vi "Test Control Experiment Dictionary.vi"() -> ()   [LabVIEW 2016]
uses:
  <userlib>/LevyLab/LV to ITX/Data/Typedefs/Dictionary--cluster.ctl
  src/Control Experiment/Control Experiment.lvclass
  <userlib>/LevyLab/LV to ITX/Data/Data.lvclass
panel:
  in  "CLOSE":bool
  out "multiple writes (ms)":u32
  out "one write (ms)":u32
  in  "TEST SPEED":bool
  in  "Append Element":cluster{"Key":string, "Value":dbl[]}
  out "Read All Items":T1[](array[typedef])
  in  "READ":bool
  in  "APPEND":bool
  in  "WRITE":bool
  in  "OK":bool
  in  "Write Element":cluster{"Key":string, "Value":dbl}
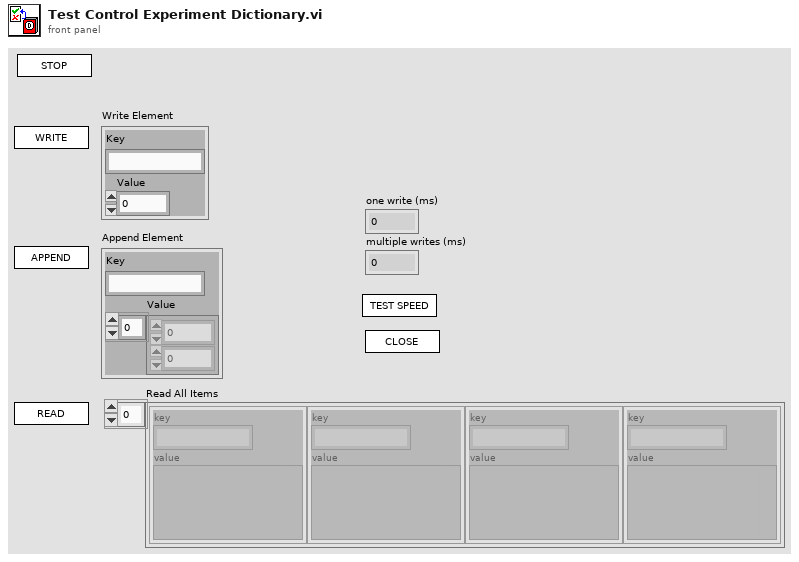
[diagram p1: front panel]
types:
  T1 = typedef "Data.lvclass/Dictionary--cluster.ctl" = cluster{"key":string, "value":variant}
  T2 = enum32{"Invalid", "Standard", "Closed", "Hidden", "Minimized", "Maximized"}
  T3 = enum32{"invalid app kind", "Development System", "Run Time System", "Student Edition", "Embedded LabVIEW", "Evaluation", "Custom"}
  T4 = cluster{"Core":cluster{"Current VI Reference":refnum<vi>, "Close Panel on Exit?":bool}, "Your Boolean data":bool, "Your string data":string, "Control Experiment.lvclass":refnum<class "Control Experiment.lvclass">}
  T5 = cluster{"Current VI Reference":refnum<vi>, "Close Panel on Exit?":bool}
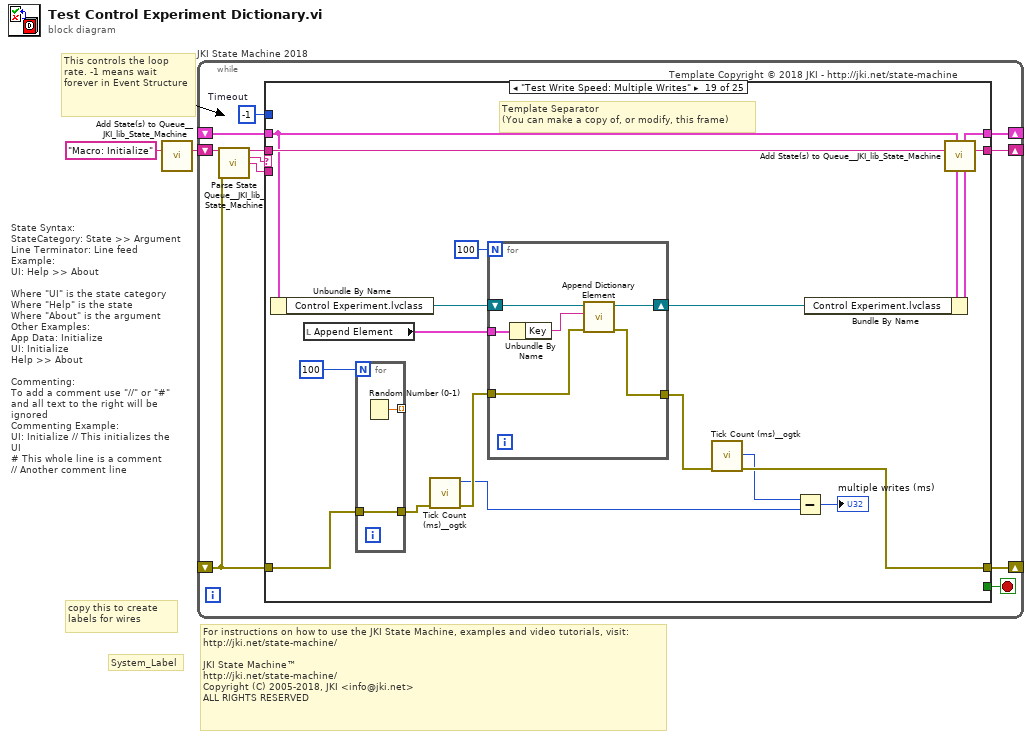
[diagram p0: block diagram]
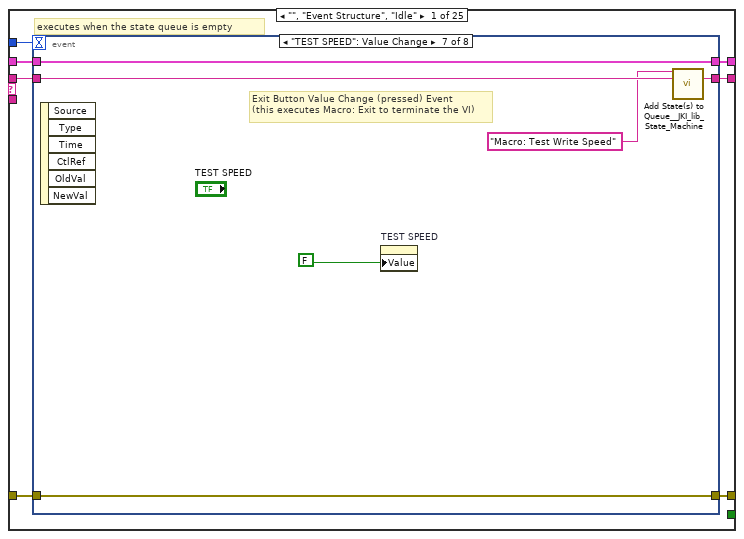
[diagram p2: hidden frame]
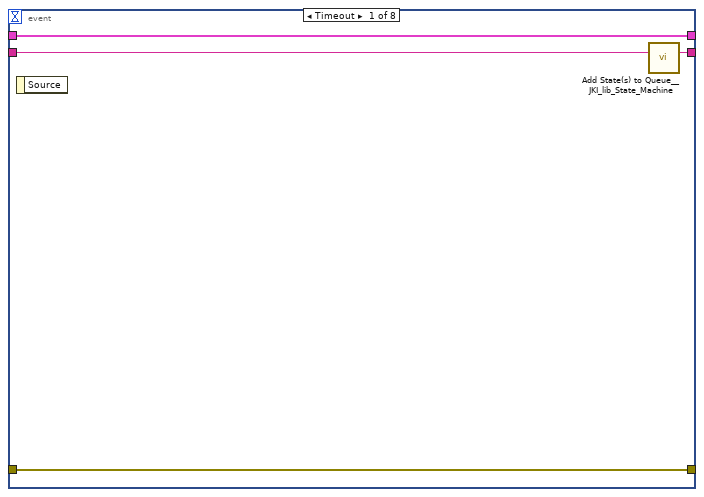
[diagram p3: hidden frame]
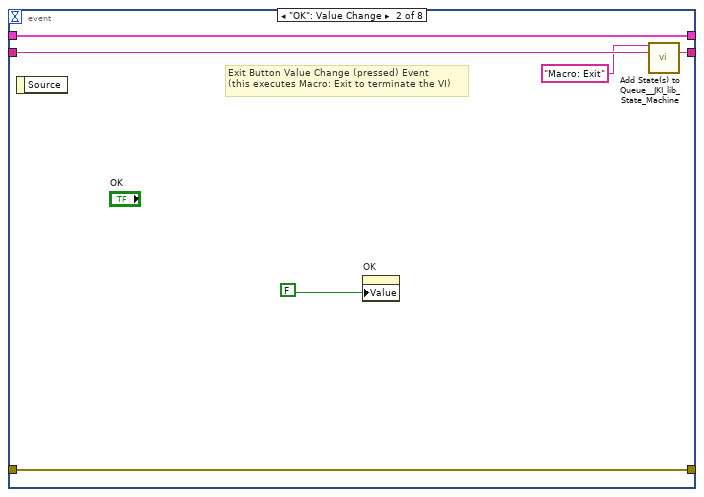
[diagram p4: hidden frame]
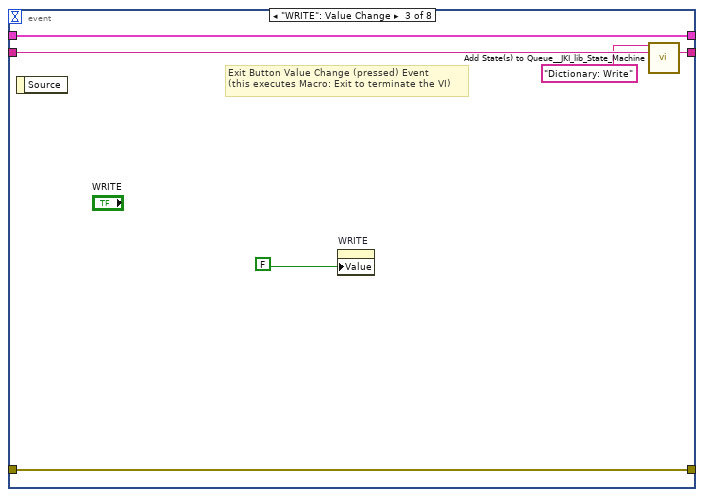
[diagram p5: hidden frame]
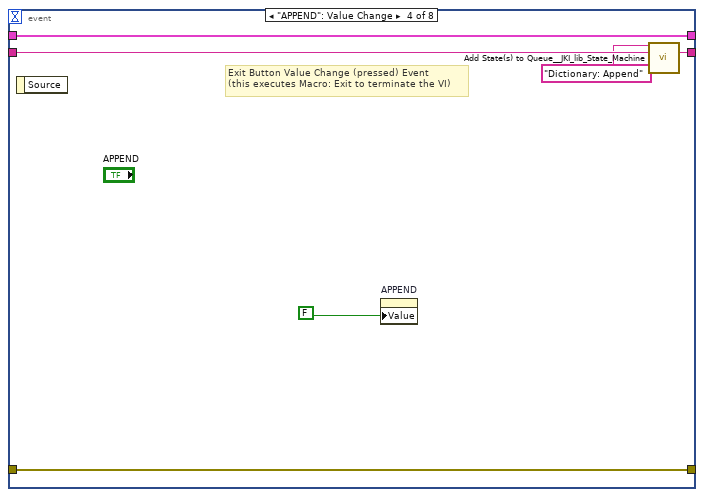
[diagram p6: hidden frame]
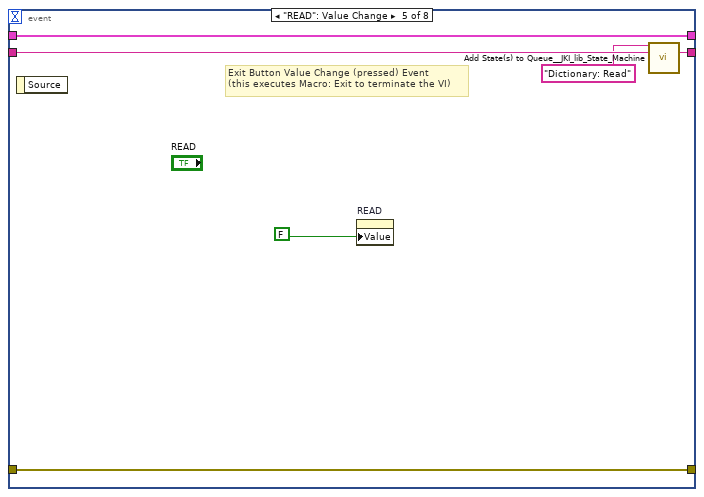
[diagram p7: hidden frame]
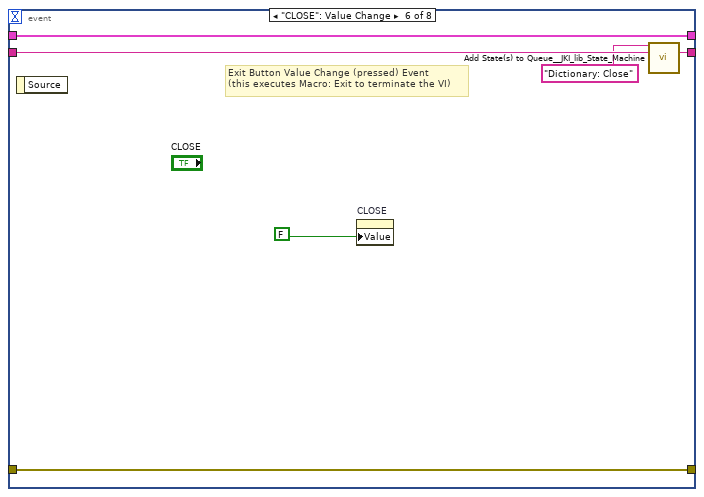
[diagram p8: hidden frame]
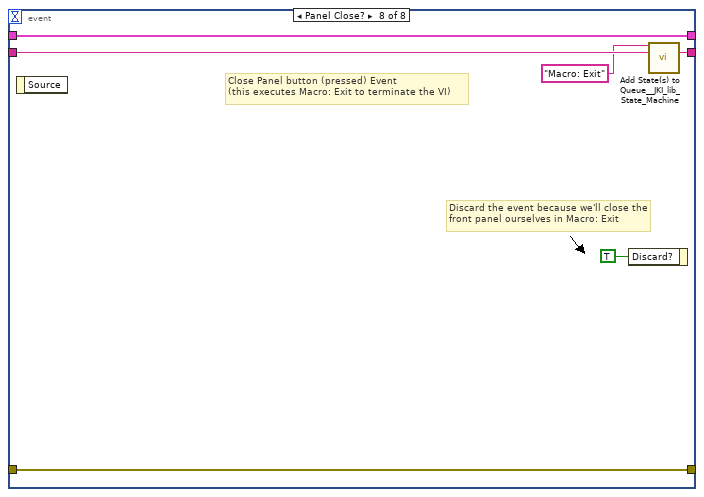
[diagram p9: hidden frame]
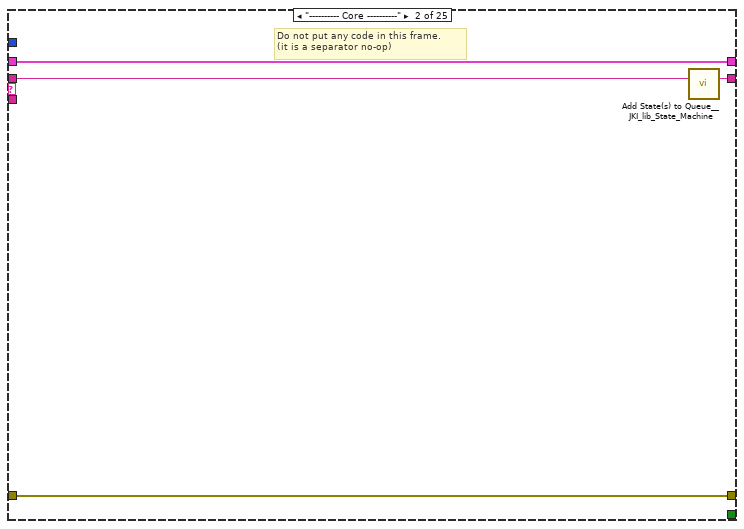
[diagram p10: hidden frame]
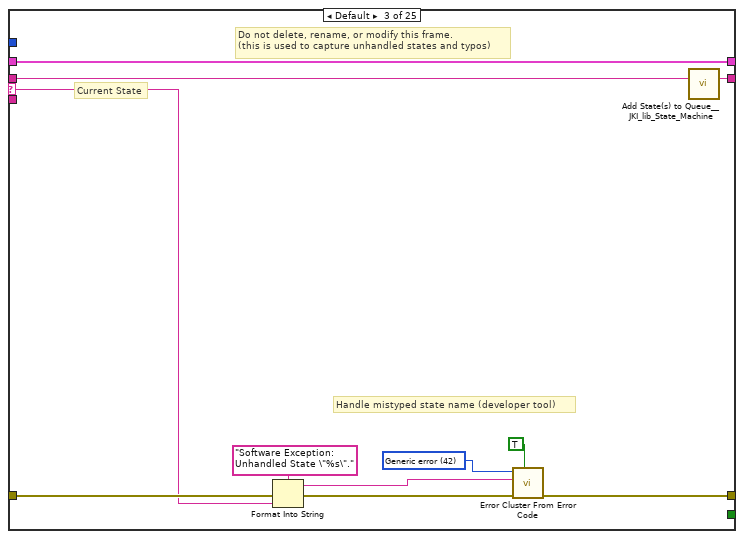
[diagram p11: hidden frame]
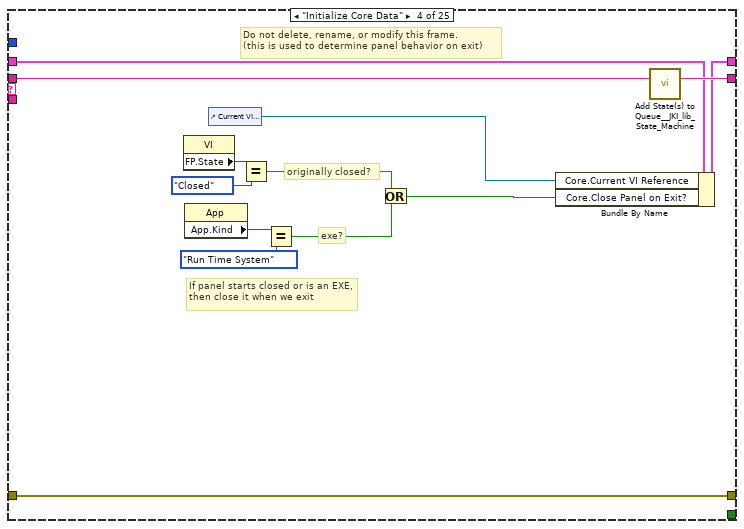
[diagram p12: hidden frame]
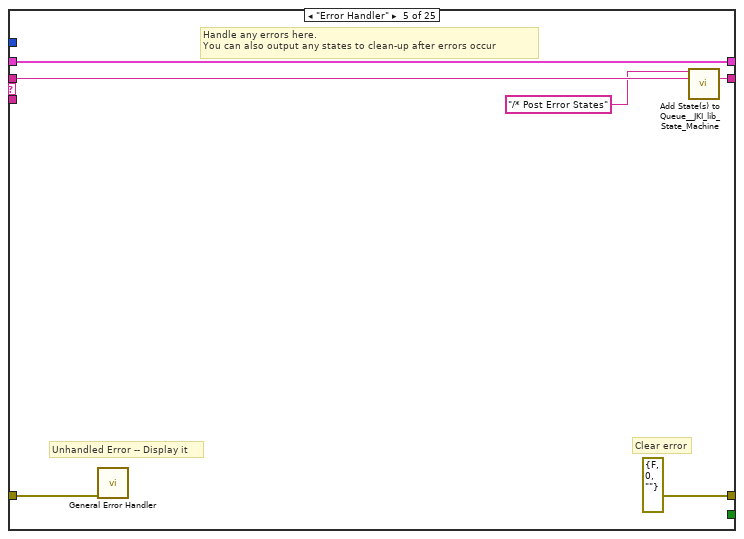
[diagram p13: hidden frame]
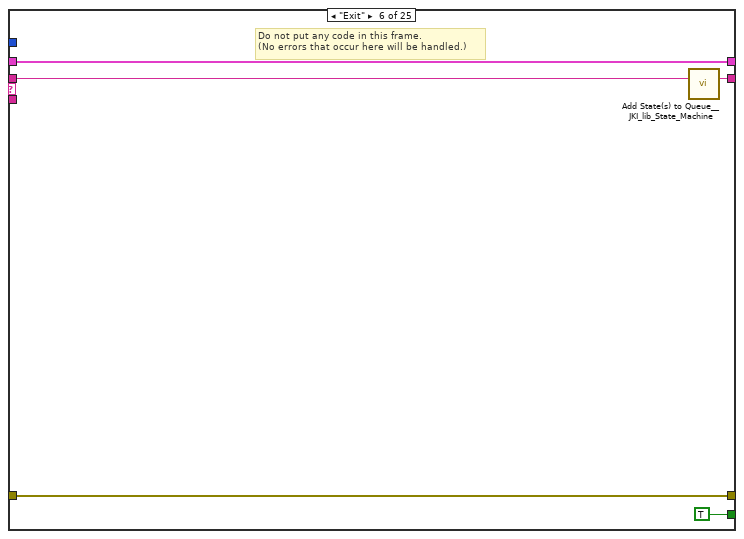
[diagram p14: hidden frame]
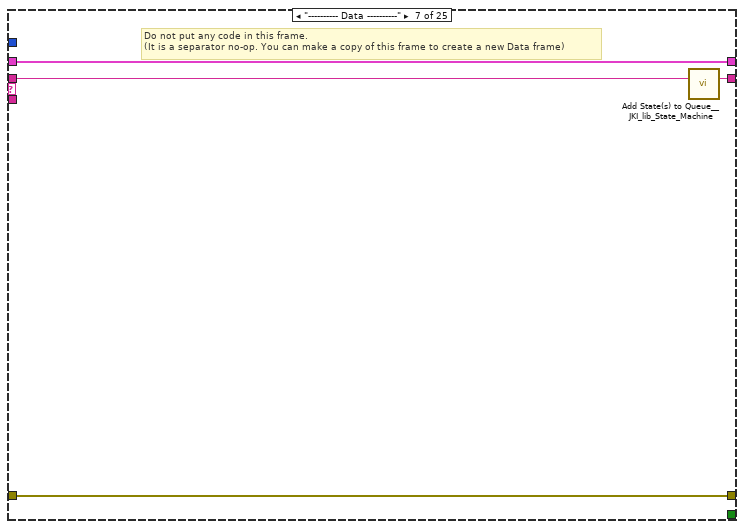
[diagram p15: hidden frame]
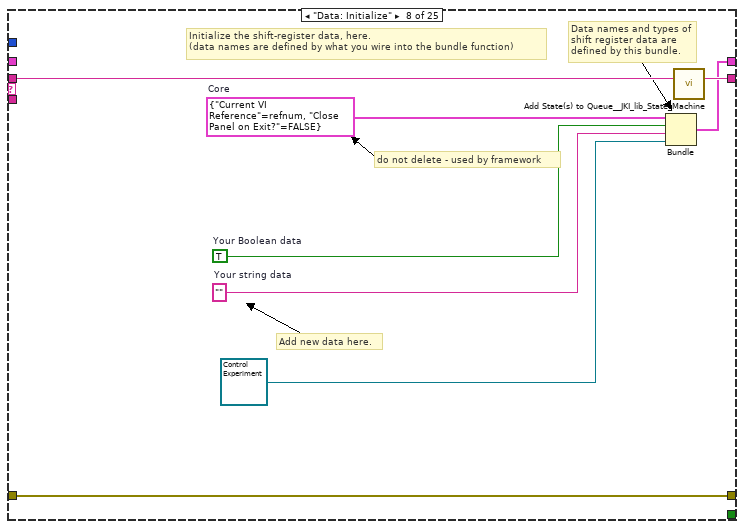
[diagram p16: hidden frame]
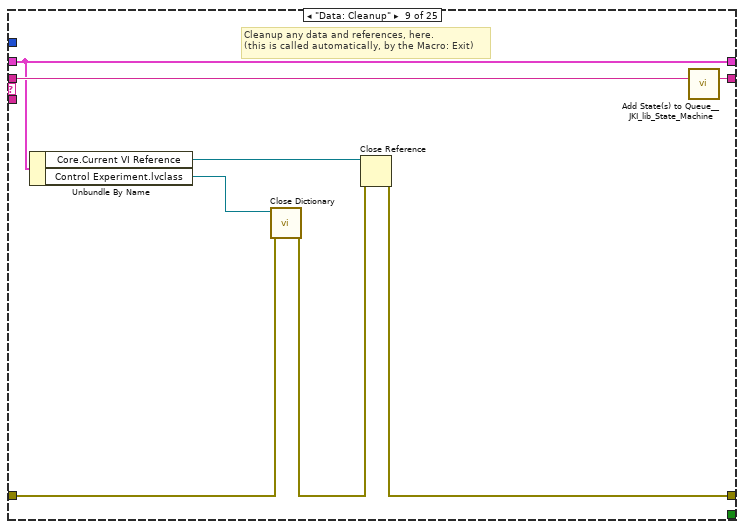
[diagram p17: hidden frame]
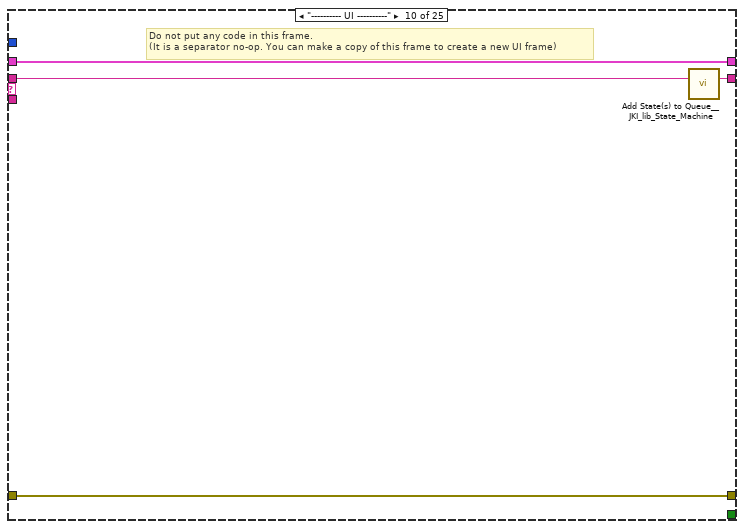
[diagram p18: hidden frame]
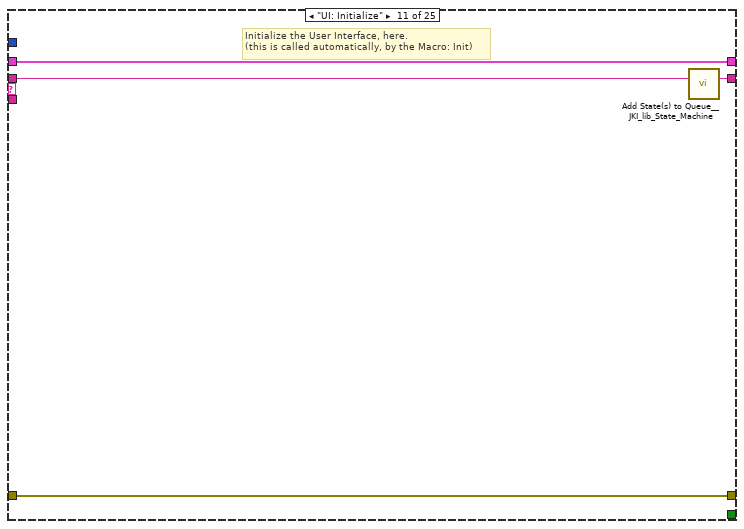
[diagram p19: hidden frame]
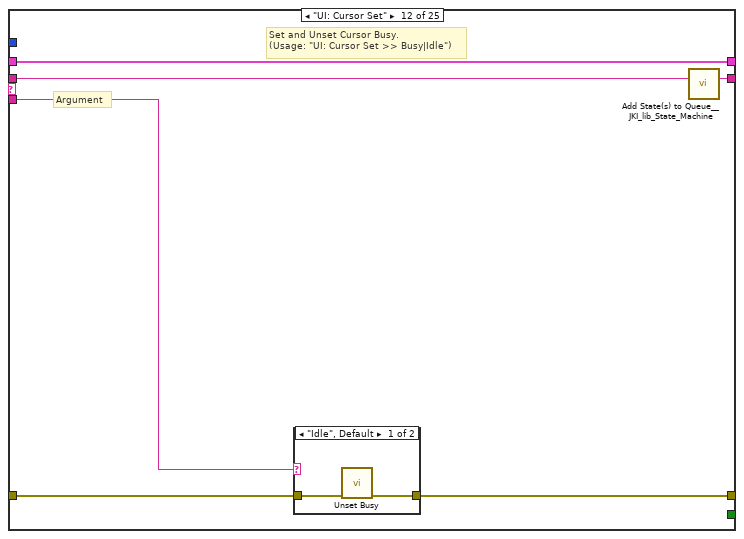
[diagram p20: hidden frame]
diagram:
  # "For instructions on how to use the JKI State Machine, examples and video tutorials, visit:\nhttp://jki.net/state-machine/\n\nJKI State Machine™\nhttp://jki.net/state-machine/\nCopyright (C) 2005-2018, JKI <info@jki.net>\nALL RIGHTS RESERVED"
  # "State Syntax:\nStateCategory: State >> Argument\nLine Terminator: Line feed\nExample:\nUI: Help >> About\n\nWhere \"UI\" is the state category\nWhere \"Help\" is the state\nWhere \"About\" is the argument\nOther Examples:\nApp Data: Initialize\nUI: Initialize\nHelp >> About\n\nCommenting:\nTo add a comment use \"//\" or \"#\" and all text to the right will be ignored\nCommenting Example:\nUI: Initialize // This initializes the UI\n# This whole line is a comment\n// Another comment line"
  # "copy this to create labels for wires"
  # "This controls the loop rate. -1 means wait forever in Event Structure"
  # "System_Label"
  n1 = call <vilib>:"Add State(s) to Queue__JKI_lib_State_Machine.vi"("State(s) in (\"\")"="Macro: Initialize") -> ("States Out"=w2:string)  [unwired: 14 in]
  n2 = while "JKI State Machine 2018" {
    shift-right: [w6] -> _
    shift-left: _ -> [w5]
    shift-right: [w9] -> _
    shift-left: _ -> [w3]
    shift-right: [w8] -> _
    shift-left: w2 -> [w10]
    stop <- w7 stop-if-true
    w4 = -1  # Timeout
    # "Template Copyright © 2018 JKI - http://jki.net/state-machine"
    n3 = call <vilib>:"Parse State Queue__JKI_lib_State_Machine.vi"("State Queue"=w10, "Error In (no error)"=w3) -> ("Remaining States"=w12:string, "Current State"=w13:string, "Arguments"=w11:string)  [unwired: 11 in]
    n4 = case shown="\"Test Write Speed: Multiple Writes\"" w13 {
      selector: w13 -> [_ _ w71 _ _ _ _ _ _ _ _ _ _ _ _ _ _ _ _ _ _ _ _ _ _]
      tunnel: w12 -> [w20 w70 w75 w94 w100 w105 w109 w117 w125 w129 w133 w139 w150 w219 w224 w229 w239 w243 w260 w286 w292 w303 w314 w323 w331]
      tunnel: w11 -> [_ _ _ _ _ _ _ _ _ _ _ w134 w144 _ _ _ _ _ _ _ _ _ _ _ _]
      tunnel: w5 -> [w18 w67 w73 w87 w97 w103 w106 _ w121 w126 w131 w137 w146 w216 w221 w226 w236 w240 w256 w282 w289 w294 w306 w316 w329]
      tunnel: [w17 w68 w77 w91 errorcluster {"status"=FALSE, "code"=0, "source"=""} ("error out") w102 w107 w114 w122 w127 w130 w135 w147 w217 w222 w227 w237 w241 w252 w279 w290 w296 w308 w318 w324] -> w9
      tunnel: w3 -> [w16 w68 w76 w91 w96 w102 w107 w114 w119 w127 w130 w136 w148 w217 w222 w227 w237 w241 w251 w270 w290 w297 w309 w319 w325]
      tunnel: [w19 w69 w74 w93 w99 w104 w108 w116 w124 w128 w132 w138 w149 w218 w223 w228 w238 w242 w259 w285 w291 w302 w313 w322 w330] -> w8
      tunnel: [_ _ _ _ _ TRUE _ _ _ _ _ _ _ _ _ _ _ _ _ _ _ _ _ _ _] -> w7
      tunnel: [w15 w67 w73 w92 w97 w103 w106 w115 w121 w126 w131 w137 w146 w216 w221 w226 w236 w240 w255 w281 w289 w293 w305 w315 w328] -> w6
      tunnel: w4 -> [w14 _ _ _ _ _ _ _ _ _ _ _ _ _ _ _ _ _ _ _ _ _ _ _ _]
      frame "", "Event Structure", "Idle" {
        # "executes when the state queue is empty"
        n5 = event shown="[6] \"TEST SPEED\": Value Change" {
          selector: _ -> [_ _ _ _ _ _ _ _]
          dyn-events: _ -> [_ _ _ _ _ _ _ _]
          timeout: w14 -> [_ _ _ _ _ _ _ _]
          tunnel: w20 -> [w24 w30 w36 w42 w48 w54 w60 w66]
          tunnel: [w23 w29 w35 w41 w47 w53 w59 w65] -> w19
          tunnel: w18 -> [w21 w27 w33 w39 w45 w51 w57 w63]
          tunnel: [w22 w28 w34 w40 w46 w52 w58 w64] -> w17
          tunnel: w16 -> [w22 w28 w34 w40 w46 w52 w58 w64]
          tunnel: [w21 w27 w33 w39 w45 w51 w57 w63] -> w15
          event Timeout {
            n6 = event-data() -> ()  [unwired: 1 in, 1 out]
            n7 = call <vilib>:"Add State(s) to Queue__JKI_lib_State_Machine.vi"("State(s) in (\"\")"=w24) -> ("States Out"=w23:string)  [unwired: 14 in]
          }
          event "OK": Value Change {
            # "Exit Button Value Change (pressed) Event\n(this executes Macro: Exit to terminate the VI)"
            n8 = event-data() -> ()  [unwired: 1 in, 1 out]
            n9 = property on="OK" class="Bool (strict)"("Value"=FALSE) -> ()  [unwired: 2 in, 2 out]
            n10 = call <vilib>:"Add State(s) to Queue__JKI_lib_State_Machine.vi"("State(s) in Front (\"\")"="Macro: Exit", "State(s) in (\"\")"=w30) -> ("States Out"=w29:string)  [unwired: 13 in]
          }
          event "WRITE": Value Change {
            # "Exit Button Value Change (pressed) Event\n(this executes Macro: Exit to terminate the VI)"
            n11 = event-data() -> ()  [unwired: 1 in, 1 out]
            n12 = property on="WRITE" class="Bool (strict)"("Value"=FALSE) -> ()  [unwired: 2 in, 2 out]
            n13 = call <vilib>:"Add State(s) to Queue__JKI_lib_State_Machine.vi"("State(s) in Front (\"\")"="Dictionary: Write", "State(s) in (\"\")"=w36) -> ("States Out"=w35:string)  [unwired: 13 in]
          }
          event "APPEND": Value Change {
            # "Exit Button Value Change (pressed) Event\n(this executes Macro: Exit to terminate the VI)"
            n14 = event-data() -> ()  [unwired: 1 in, 1 out]
            n15 = property on="APPEND" class="Bool (strict)"("Value"=FALSE) -> ()  [unwired: 2 in, 2 out]
            n16 = call <vilib>:"Add State(s) to Queue__JKI_lib_State_Machine.vi"("State(s) in Front (\"\")"="Dictionary: Append", "State(s) in (\"\")"=w42) -> ("States Out"=w41:string)  [unwired: 13 in]
          }
          event "READ": Value Change {
            # "Exit Button Value Change (pressed) Event\n(this executes Macro: Exit to terminate the VI)"
            n17 = event-data() -> ()  [unwired: 1 in, 1 out]
            n18 = property on="READ" class="Bool (strict)"("Value"=FALSE) -> ()  [unwired: 2 in, 2 out]
            n19 = call <vilib>:"Add State(s) to Queue__JKI_lib_State_Machine.vi"("State(s) in Front (\"\")"="Dictionary: Read", "State(s) in (\"\")"=w48) -> ("States Out"=w47:string)  [unwired: 13 in]
          }
          event "CLOSE": Value Change {
            # "Exit Button Value Change (pressed) Event\n(this executes Macro: Exit to terminate the VI)"
            n20 = event-data() -> ()  [unwired: 1 in, 1 out]
            n21 = property on="CLOSE" class="Bool (strict)"("Value"=FALSE) -> ()  [unwired: 2 in, 2 out]
            n22 = call <vilib>:"Add State(s) to Queue__JKI_lib_State_Machine.vi"("State(s) in Front (\"\")"="Dictionary: Close", "State(s) in (\"\")"=w54) -> ("States Out"=w53:string)  [unwired: 13 in]
          }
          event "TEST SPEED": Value Change {
            # "Exit Button Value Change (pressed) Event\n(this executes Macro: Exit to terminate the VI)"
            n23 = event-data() -> ()  [unwired: 1 in, 6 out]
            n24 = property on="TEST SPEED" class="Bool (strict)"("Value"=FALSE) -> ()  [unwired: 2 in, 2 out]
            n25 = call <vilib>:"Add State(s) to Queue__JKI_lib_State_Machine.vi"("State(s) in Front (\"\")"="Macro: Test Write Speed", "State(s) in (\"\")"=w60) -> ("States Out"=w59:string)  [unwired: 13 in]
          }
          event Panel Close? {
            # "Discard the event because we'll close the front panel ourselves in Macro: Exit"
            # "Close Panel button (pressed) Event\n(this executes Macro: Exit to terminate the VI)"
            n26 = event-data() -> ()  [unwired: 1 in, 1 out]
            n27 = event-data("Discard?"=TRUE) -> ()  [unwired: 1 in, 1 out]
            n28 = call <vilib>:"Add State(s) to Queue__JKI_lib_State_Machine.vi"("State(s) in Front (\"\")"="Macro: Exit", "State(s) in (\"\")"=w66) -> ("States Out"=w65:string)  [unwired: 13 in]
          }
        }
      }
      frame "---------- Core ----------" {
        # "Do not put any code in this frame.\n(it is a separator no-op)"
        n29 = call <vilib>:"Add State(s) to Queue__JKI_lib_State_Machine.vi"("State(s) in (\"\")"=w70) -> ("States Out"=w69:string)  [unwired: 14 in]
      }
      frame Default {
        w80 = 42 items=["No error", "Argument error", "Memory is full", "Out of zone", "End of file", "File already open", "Generic file I/O error", "File not found", "File permission error", "Disk is full", "Duplicate path", "Too many files open", "System feature not enabled", "Resource file not found", "Cannot add resource", "Resource not found", "Image not found", "Image memory error", "Pen does not exist", "Config type invalid", "Config token not found", "Config parse error", "Config memory error", "Bad external code format", "Bad external code offset", "External code not present", "Null window", "Destroy window error", "Null menu", "Print aborted", "Bad print record", "Print driver error", "Windows error during printing", "Memory error during printing", "Print dialog error", "Generic print error", "Invalid device refnum", "Device not found", "Device parameter error", "Device unit error", "Cannot open device", "Device call aborted", "Generic error", "Cancelled by user", "Object ID too low", "Object ID too high", "Object not in heap", "Unknown heap", "Unknown object (invalid DefProc)", "Unknown object (DefProc not in table)", "Message out of range", "Invalid (null) method", "Unknown message", "Manager call not supported", "Bad address", "Network operation in progress", "Network operation timed out", "Connection is busy", "Network attribute not supported", "Network error", "Address in use", "System out of memory", "Connection aborted", "Connection refused", "Not connected", "Already connected", "Connection closed", "Initialization error (interapplication manager)", "Bad occurrence", "Wait on unbound occurrence handler", "Occurrence queue overflow", "Datalog type conflict", "Unused", "Unrecognized type (interapplication manager)", "Memory corrupt", "Failed to make temporary DLL", "Old CIN version", "Drag socket not found", "Failed to load drop-object", "Failed to register OLE object", "Failed to release OLE object", "Format specifier type mismatch", "Unknown format specifier", "Too few format specifiers", "Too many format specifiers", "Scan failed", "Newer CIN version", "Error converting to variant", "Runtime menu error", "Password tampered", "Variant attribute not found", "Incompatible variant data type", "Event data is not available", "Event Store is not present", "Occurrence is not found", "Event Queue is not created", "Event info is not available", "Refnum passed is NULL", "Error retrieving Class GUID", "Error retrieving CoClass GUID", "Error retrieving TypeLib GUID.", "Bad built application magic bytes.", "Specific driver is different from the specific driver associated with the Logical Name.", "There is no session opened to the class driver.", "Max Error", "MAX - Error with config objects", "MAX - Error loading configuration", "MAX - Group not supported"]
        # "Current State"
        # "Do not delete, rename, or modify this frame.\n(this is used to capture unhandled states and typos)"
        # "Handle mistyped state name (developer tool)"
        n30 = Format Into String(format string="Software Exception: Unhandled State \"%s\"." ("message"), error in=w76, w71) -> (resulting string=w79:string, error out=w78:errorcluster)  [unwired: 1 in]
        n31 = call <vilib>:"Error Cluster From Error Code.vi"("show call chain? (False)"=TRUE, "error in (no error)"=w78, "error message (\"\")"=w79, "error code (0)"=w80) -> ("error out"=w77:errorcluster)  [unwired: 5 in]
        n32 = call <vilib>:"Add State(s) to Queue__JKI_lib_State_Machine.vi"("State(s) in (\"\")"=w75) -> ("States Out"=w74:string)  [unwired: 14 in]
      }
      frame "Initialize Core Data" {
        # "Do not delete, rename, or modify this frame.\n(this is used to determine panel behavior on exit)"
        # "originally closed?"
        # "exe?"
        # "If panel starts closed or is an EXE, then close it when we exit"
        n33 = property class="VI"() -> ("FP.State"=w84:T2)  [unwired: 2 in, 2 out]
        n34 = property class="App"() -> ("App.Kind"=w90:T3)  [unwired: 2 in, 2 out]
        n35 = control-ref of="Current VI Reference"() -> (w85:refnum<vi>)
        n36 = Equal?(x=w84, y=T2."Closed" ("Front Panel Window:State")) -> (x = y?=w82:bool)
        n37 = Equal?(x=w90, y=T3."Run Time System" ("Application:Kind")) -> (x = y?=w88:bool)
        n38 = Or(x=w82, y=w88) -> (x .or. y?=w86:bool)
        n39 = Bundle By Name(cluster=w87, "Core.Current VI Reference"=w85, "Core.Close Panel on Exit?"=w86) -> (w92:T4)
        n40 = call <vilib>:"Add State(s) to Queue__JKI_lib_State_Machine.vi"("State(s) in (\"\")"=w94) -> ("States Out"=w93:string)  [unwired: 14 in]
      }
      frame "Error Handler" {
        # "Unhandled Error -- Display it"
        # "Handle any errors here.\nYou can also output any states to clean-up after errors occur"
        # "Clear error"
        n41 = call <vilib>:"General Error Handler.vi"("error in (no error)"=w96) -> ()  [unwired: 10 in, 5 out]
        n42 = call <vilib>:"Add State(s) to Queue__JKI_lib_State_Machine.vi"("State(s) in Front (\"\")"="/* Post Error States", "State(s) in (\"\")"=w100) -> ("States Out"=w99:string)  [unwired: 13 in]
      }
      frame "Exit" {
        # "Do not put any code in this frame.\n(No errors that occur here will be handled.)"
        n43 = call <vilib>:"Add State(s) to Queue__JKI_lib_State_Machine.vi"("State(s) in (\"\")"=w105) -> ("States Out"=w104:string)  [unwired: 14 in]
      }
      frame "---------- Data ----------" {
        # "Do not put any code in this frame.\n(It is a separator no-op. You can make a copy of this frame to create a new Data frame)"
        n44 = call <vilib>:"Add State(s) to Queue__JKI_lib_State_Machine.vi"("State(s) in (\"\")"=w109) -> ("States Out"=w108:string)  [unwired: 14 in]
      }
      frame "Data: Initialize" {
        w111 = T5 {"Current VI Reference"=refnum, "Close Panel on Exit?"=FALSE}  # Core
        w113 = TRUE  # Your Boolean data
        w112 = ""  # Your string data
        # "do not delete - used by framework"
        # "Add new data here."
        # "Data names and types of shift register data are defined by this bundle."
        # "Initialize the shift-register data, here.\n(data names are defined by what you wire into the bundle function)"
        n45 = Bundle("Core"=w111, "Your Boolean data"=w113, "Your string data"=w112, "Control Experiment.lvclass"=refnum<class "Control Experiment.lvclass"> refnum) -> (w115:T4)  [unwired: 1 in]
        n46 = call <vilib>:"Add State(s) to Queue__JKI_lib_State_Machine.vi"("State(s) in (\"\")"=w117) -> ("States Out"=w116:string)  [unwired: 14 in]
      }
      frame "Data: Cleanup" {
        # "Cleanup any data and references, here.\n(this is called automatically, by the Macro: Exit)"
        n47 = Unbundle By Name(w121) -> ("Core.Current VI Reference"=w123:refnum<vi>, "Control Experiment.lvclass"=w120:refnum<class "Control Experiment.lvclass">)
        n48 = call "Close Dictionary.vi"("error in (no error)"=w119, "Control Experiment in"=w120) -> ("error out"=w118:errorcluster)  [unwired: 8 in, 1 out]
        n49 = Close Reference(reference=w123, error in (no error)=w118) -> (error out=w122:errorcluster)
        n50 = call <vilib>:"Add State(s) to Queue__JKI_lib_State_Machine.vi"("State(s) in (\"\")"=w125) -> ("States Out"=w124:string)  [unwired: 14 in]
      }
      frame "---------- UI ----------" {
        # "Do not put any code in this frame.\n(It is a separator no-op. You can make a copy of this frame to create a new UI frame)"
        n51 = call <vilib>:"Add State(s) to Queue__JKI_lib_State_Machine.vi"("State(s) in (\"\")"=w129) -> ("States Out"=w128:string)  [unwired: 14 in]
      }
      frame "UI: Initialize" {
        # "Initialize the User Interface, here.\n(this is called automatically, by the Macro: Init)"
        n52 = call <vilib>:"Add State(s) to Queue__JKI_lib_State_Machine.vi"("State(s) in (\"\")"=w133) -> ("States Out"=w132:string)  [unwired: 14 in]
      }
      frame "UI: Cursor Set" {
        # "Argument"
        # "Set and Unset Cursor Busy.\n(Usage: \"UI: Cursor Set >> Busy|Idle\")"
        n53 = case shown="\"Idle\", Default" w134 {
          tunnel: w136 -> [w141 w143]
          tunnel: [w140 w142] -> w135
          frame "Idle", Default {
            n54 = call <vilib>:"Unset Busy.vi"("error in (no error)"=w141) -> ("error out"=w140:errorcluster)  [unwired: 10 in]
          }
          frame "Busy" {
            n55 = call <vilib>:"Set Busy.vi"("error in (no error)"=w143) -> ("error out"=w142:errorcluster)  [unwired: 9 in, 1 out]
          }
        }
        n56 = call <vilib>:"Add State(s) to Queue__JKI_lib_State_Machine.vi"("State(s) in (\"\")"=w139) -> ("States Out"=w138:string)  [unwired: 14 in]
      }
      frame "UI: Front Panel State" {
        # "Argument"
        # "Set Front Panel Open or Closed\n(Usage: \"UI: Front Panel State >> Open|Close\")"
        n57 = Unbundle By Name(w146) -> ("Core.Current VI Reference"=w145:refnum<vi>)
        n58 = case shown="\"Minimize\", \"Minimized\"" w144 {
          tunnel: w148 -> [w156 w171 w182 w195 w208]
          tunnel: [w158 w172 w184 w197 w210] -> w147
          tunnel: w145 -> [w157 w169 w183 w196 w209]
          frame "Open", "Standard", Default {
            w151 = T2."Standard" ("State")
            n59 = property class="VI"(reference=w157, error in=w156) -> (reference out=w154:refnum<vi>, error out=w155:errorcluster, "FP.State"=w153:T2)
            n60 = Not Equal?(x=w153, y=w151) -> (x != y?=w152:bool)
            n61 = case shown="True" w152 {
              tunnel: [w162 w164] -> w158
              tunnel: w155 -> [w161 w164]
              tunnel: w154 -> [w160 _]
              tunnel: w151 -> [w159 _]
              frame True {
                n62 = invoke class="VI" method="FP.Open"(reference=w160, error in=w161, "Activate"=TRUE, "State"=w159) -> (error out=w162:errorcluster)  [unwired: 1 in, 4 out]
              }
              frame False {
              }
            }
          }
          frame "Close", "Closed" {
            n63 = property class="VI"(reference=w169, error in=w171) -> (reference out=w168:refnum<vi>, error out=w170:errorcluster, "FP.State"=w166:T2)
            n64 = Not Equal?(x=w166, y=T2."Closed" ("Front Panel Window:State")) -> (x != y?=w165:bool)
            n65 = case shown="True" w165 {
              tunnel: [w173 w176] -> w172
              tunnel: w170 -> [w173 w175]
              tunnel: w168 -> [_ w174]
              frame False {
              }
              frame True {
                n66 = invoke class="VI" method="FP.Close"(reference=w174, error in=w175) -> (error out=w176:errorcluster)  [unwired: 1 in, 2 out]
              }
            }
          }
          frame "Hidden", "Hide" {
            w177 = T2."Hidden" ("State")
            n67 = property class="VI"(reference=w183, error in=w182) -> (reference out=w180:refnum<vi>, error out=w181:errorcluster, "FP.State"=w179:T2)
            n68 = Not Equal?(x=w179, y=w177) -> (x != y?=w178:bool)
            n69 = case shown="True" w178 {
              tunnel: [w188 w189] -> w184
              tunnel: w181 -> [w187 w189]
              tunnel: w180 -> [w186 _]
              tunnel: w177 -> [w185 _]
              frame True {
                n70 = invoke class="VI" method="FP.Open"(reference=w186, error in=w187, "State"=w185) -> (error out=w188:errorcluster)  [unwired: 2 in, 4 out]
              }
              frame False {
              }
            }
          }
          frame "Minimize", "Minimized" {
            w190 = T2."Minimized" ("State")
            n71 = property class="VI"(reference=w196, error in=w195) -> (reference out=w193:refnum<vi>, error out=w194:errorcluster, "FP.State"=w192:T2)
            n72 = Not Equal?(x=w192, y=w190) -> (x != y?=w191:bool)
            n73 = case shown="True" w191 {
              tunnel: [w201 w202] -> w197
              tunnel: w194 -> [w200 w202]
              tunnel: w193 -> [w199 _]
              tunnel: w190 -> [w198 _]
              frame True {
                n74 = invoke class="VI" method="FP.Open"(reference=w199, error in=w200, "State"=w198) -> (error out=w201:errorcluster)  [unwired: 2 in, 4 out]
              }
              frame False {
              }
            }
          }
          frame "Maximize", "Maximized" {
            w203 = T2."Maximized" ("State")
            n75 = property class="VI"(reference=w209, error in=w208) -> (reference out=w206:refnum<vi>, error out=w207:errorcluster, "FP.State"=w205:T2)
            n76 = Not Equal?(x=w205, y=w203) -> (x != y?=w204:bool)
            n77 = case shown="True" w204 {
              tunnel: [w214 w215] -> w210
              tunnel: w207 -> [w213 w215]
              tunnel: w206 -> [w212 _]
              tunnel: w203 -> [w211 _]
              frame True {
                n78 = invoke class="VI" method="FP.Open"(reference=w212, error in=w213, "State"=w211) -> (error out=w214:errorcluster)  [unwired: 2 in, 4 out]
              }
              frame False {
              }
            }
          }
        }
        n79 = call <vilib>:"Add State(s) to Queue__JKI_lib_State_Machine.vi"("State(s) in (\"\")"=w150) -> ("States Out"=w149:string)  [unwired: 14 in]
      }
      frame "---------- Macro ----------" {
        # "Do not put any code in this frame.\n(It is a separator no-op. You can make a copy of this frame to create a new Macro frame)"
        n80 = call <vilib>:"Add State(s) to Queue__JKI_lib_State_Machine.vi"("State(s) in (\"\")"=w219) -> ("States Out"=w218:string)  [unwired: 14 in]
      }
      frame "Macro: Initialize" {
        w220 = "Data: Initialize\nInitialize Core Data\nUI: Initialize\nUI: Front Panel State >> Open"  # Data: Initialize Initialize Core Data UI: Initialize UI: Front Panel State >> Open
        # "Initialization Macro\n(This is called once, when the VI starts)"
        n81 = call <vilib>:"Add State(s) to Queue__JKI_lib_State_Machine.vi"("State(s) in Front (\"\")"=w220, "State(s) in (\"\")"=w224) -> ("States Out"=w223:string)  [unwired: 13 in]
      }
      frame "Macro: Test Write Speed" {
        # "Initialization Macro\n(This is called once, when the VI starts)"
        n82 = call <vilib>:"Add State(s) to Queue__JKI_lib_State_Machine.vi"("State(s) in Front (\"\")"="Test Write Speed: Multiple Writes\nDictionary: Read\nTest Write Speed: One Write\nDictionary: Read", "State(s) in (\"\")"=w229) -> ("States Out"=w228:string)  [unwired: 13 in]
      }
      frame "Macro: Exit" {
        # "Exit Macro\n(This is called once, when the VI exits)"
        n83 = Unbundle By Name(w236) -> ("Core.Close Panel on Exit?"=w235:bool)
        n84 = Select(t="UI: Front Panel State >> Close", s=w235, f="") -> (s? t:f=w232:string)
        n85 = call <vilib>:"Add State(s) to Queue__JKI_lib_State_Machine.vi"("State(s) in (\"\")"=w232, "State(s) at Back (\"\")"="Data: Cleanup\nExit") -> ("States Out"=w230:string)  [unwired: 13 in]
        n86 = call <vilib>:"Add State(s) to Queue__JKI_lib_State_Machine.vi"("State(s) in Front (\"\")"=w230, "State(s) in (\"\")"=w239) -> ("States Out"=w238:string)  [unwired: 13 in]
      }
      frame "---------- Test Write Speed ----------" {
        # "Do not put any code in this frame.\n(It is a separator no-op. You can make a copy of this frame to create a new Macro frame)"
        n87 = call <vilib>:"Add State(s) to Queue__JKI_lib_State_Machine.vi"("State(s) in (\"\")"=w243) -> ("States Out"=w242:string)  [unwired: 14 in]
      }
      frame "Test Write Speed: Multiple Writes" {
        # "Template Separator\n(You can make a copy of, or modify, this frame)"
        n88 = Unbundle By Name(w256) -> ("Control Experiment.lvclass"=w258:refnum<class "Control Experiment.lvclass">)
        n89 = local read "Append Element"() -> (w254:cluster{"Key":string, "Value":dbl[]})
        n90 = for {
          N: 100 -> [_]
          tunnel: [w262] -> _ mode=indexing
          tunnel: [w261] -> w250
          tunnel: w251 -> [w261]
          n91 = Random Number (0-1)() -> (number: 0 to 1=w262:dbl)
        }
        n92 = call <userlib>:"Tick Count (ms)__ogtk.vi"("error in (no error)"=w250) -> ("error out"=w253:errorcluster, "millisecond timer value"=w247:u32)  [unwired: 9 in]
        n93 = for {
          N: 100 -> [_]
          tunnel: w254 -> [w266]
          tunnel: w253 -> [w264]
          tunnel: [w263] -> w249
          shift-right: [w267] -> w257
          shift-left: w258 -> [w268]
          n94 = Unbundle By Name(w266) -> ("Key"=w265:string)
          n95 = call "Append Dictionary Element.vi"("error in (no error)"=w264, "key"=w265, "Control Experiment in"=w268) -> ("error out"=w263:errorcluster, "Control Experiment out"=w267:refnum<class "Control Experiment.lvclass">)  [unwired: 7 in]
        }
        n96 = call <userlib>:"Tick Count (ms)__ogtk.vi"("error in (no error)"=w249) -> ("error out"=w252:errorcluster, "millisecond timer value"=w248:u32)  [unwired: 9 in]
        n97 = Subtract(x=w248, y=w247) -> (x-y=→"multiple writes (ms)":u32)
        n98 = Bundle By Name(cluster=w256, "Control Experiment.lvclass"=w257) -> (w255:T4)
        n99 = call <vilib>:"Add State(s) to Queue__JKI_lib_State_Machine.vi"("State(s) in (\"\")"=w260) -> ("States Out"=w259:string)  [unwired: 14 in]
      }
      frame "Test Write Speed: One Write" {
        # "Template Separator\n(You can make a copy of, or modify, this frame)"
        n100 = Unbundle By Name(w282) -> ("Control Experiment.lvclass"=w284:refnum<class "Control Experiment.lvclass">)
        n101 = local read "Append Element"() -> (w280:cluster{"Key":string, "Value":dbl[]})
        n102 = for {
          N: 10000 -> [_]
          tunnel: [w288] -> w271 mode=indexing
          tunnel: [w287] -> w269
          tunnel: w270 -> [w287]
          n103 = Random Number (0-1)() -> (number: 0 to 1=w288:dbl)
        }
        n104 = call <userlib>:"Tick Count (ms)__ogtk.vi"("error in (no error)"=w269) -> ("error out"=w276:errorcluster, "millisecond timer value"=w273:u32)  [unwired: 9 in]
        n105 = Unbundle By Name(w280) -> ("Key"=w278:string)
        n106 = call "Append Dictionary Element.vi"("error in (no error)"=w276, "value"=w271, "key"=w278, "Control Experiment in"=w284) -> ("error out"=w275:errorcluster, "Control Experiment out"=w283:refnum<class "Control Experiment.lvclass">)  [unwired: 6 in]
        n107 = call <userlib>:"Tick Count (ms)__ogtk.vi"("error in (no error)"=w275) -> ("error out"=w279:errorcluster, "millisecond timer value"=w274:u32)  [unwired: 9 in]
        n108 = Subtract(x=w274, y=w273) -> (x-y=→"one write (ms)":u32)
        n109 = Bundle By Name(cluster=w282, "Control Experiment.lvclass"=w283) -> (w281:T4)
        n110 = call <vilib>:"Add State(s) to Queue__JKI_lib_State_Machine.vi"("State(s) in (\"\")"=w286) -> ("States Out"=w285:string)  [unwired: 14 in]
      }
      frame "---------- Dictionary ----------" {
        # "Template Separator\n(You can make a copy of, or modify, this frame)"
        n111 = call <vilib>:"Add State(s) to Queue__JKI_lib_State_Machine.vi"("State(s) in (\"\")"=w292) -> ("States Out"=w291:string)  [unwired: 14 in]
      }
      frame "Dictionary: Write" {
        # "Your code here.\n(You can make a copy of, or modify, this frame)"
        n112 = Unbundle By Name(w294) -> ("Control Experiment.lvclass"=w298:refnum<class "Control Experiment.lvclass">)
        n113 = Unbundle By Name("Write Element") -> ("Key"=w300:string, "Value"=w299:dbl)
        n114 = call "Write Dictionary Element.vi"("error in (no error)"=w297, "value"=w299, "key"=w300, "Control Experiment in"=w298) -> ("error out"=w296:errorcluster, "Control Experiment out"=w295:refnum<class "Control Experiment.lvclass">)  [unwired: 6 in]
        n115 = Bundle By Name(cluster=w294, "Control Experiment.lvclass"=w295) -> (w293:T4)
        n116 = call <vilib>:"Add State(s) to Queue__JKI_lib_State_Machine.vi"("State(s) in (\"\")"=w303) -> ("States Out"=w302:string)  [unwired: 14 in]
      }
      frame "Dictionary: Append" {
        # "Your code here.\n(You can make a copy of, or modify, this frame)"
        n117 = Unbundle By Name(w306) -> ("Control Experiment.lvclass"=w310:refnum<class "Control Experiment.lvclass">)
        n118 = Unbundle By Name("Append Element") -> ("Key"=w311:string, "Value"=w312:dbl[])
        n119 = call "Append Dictionary Element.vi"("error in (no error)"=w309, "value"=w312, "key"=w311, "Control Experiment in"=w310) -> ("error out"=w308:errorcluster, "Control Experiment out"=w307:refnum<class "Control Experiment.lvclass">)  [unwired: 6 in]
        n120 = Bundle By Name(cluster=w306, "Control Experiment.lvclass"=w307) -> (w305:T4)
        n121 = call <vilib>:"Add State(s) to Queue__JKI_lib_State_Machine.vi"("State(s) in (\"\")"=w314) -> ("States Out"=w313:string)  [unwired: 14 in]
      }
      frame "Dictionary: Read" {
        # "Template Separator\n(You can make a copy of, or modify, this frame)"
        n122 = Unbundle By Name(w316) -> ("Control Experiment.lvclass"=w321:refnum<class "Control Experiment.lvclass">)
        n123 = call "Read All Dictionary Elements.vi"("error in (no error)"=w319, "Control Experiment in"=w321) -> ("error out"=w318:errorcluster, "items"=→"Read All Items":T1[], "Control Experiment out"=w317:refnum<class "Control Experiment.lvclass">)  [unwired: 7 in]
        n124 = Bundle By Name(cluster=w316, "Control Experiment.lvclass"=w317) -> (w315:T4)
        n125 = call <vilib>:"Add State(s) to Queue__JKI_lib_State_Machine.vi"("State(s) in (\"\")"=w323) -> ("States Out"=w322:string)  [unwired: 14 in]
      }
      frame "Dictionary: Close" {
        # "Template Separator\n(You can make a copy of, or modify, this frame)"
        n126 = Unbundle By Name(w329) -> ("Control Experiment.lvclass"=w327:refnum<class "Control Experiment.lvclass">)
        n127 = call "Close Dictionary.vi"("error in (no error)"=w325, "Control Experiment in"=w327) -> ("error out"=w324:errorcluster, "Control Experiment out"=w326:refnum<class "Control Experiment.lvclass">)  [unwired: 8 in]
        n128 = Bundle By Name(cluster=w329, "Control Experiment.lvclass"=w326) -> (w328:T4)
        n129 = call <vilib>:"Add State(s) to Queue__JKI_lib_State_Machine.vi"("State(s) in (\"\")"=w331) -> ("States Out"=w330:string)  [unwired: 14 in]
      }
    }
  }
